vi "BrushedData (RT).vi"() -> ()   [LabVIEW 2013]
uses:
  <vilib>/FPGAPlugInAG/sbRIO-9626/niLvFpga_Open_sbRIO-9626.vi
  <vilib>/rvi/interface/common/dynamic/niFpgaDynamicAddResources.vi
  <vilib>/FPGAPlugInAG/Dynamic/niLvFpga_Reset_Dynamic.vi
  <vilib>/FPGAPlugInAG/Dynamic/niLvFpga_Run_Dynamic.vi
  <vilib>/rvi/interface/common/niFpgaWaitOnOcc.vi
  <vilib>/Utility/error.llb/Error Cluster From Error Code.vi
  <vilib>/rvi/errors/niLvFpgaAdjustHostInterfaceError.vi
  <vilib>/rvi/interface/nirviOpenFPGA/nirviOpenFPGA.xnode
  FPGA/bitfiles/TI sbRIO PWM (FPGA) v1.0.lvbitx
  <vilib>/rvi/interface/nirviMethod/nirviMethod.xnode
  <vilib>/rvi/interface/nirviReadWriteControl/nirviReadWriteControl.xnode
  <vilib>/FPGAPlugInAG/Dynamic/niLvFpga_ReadFifo_Dynamic.vi
  <vilib>/rvi/errors/niLvFpgaMergeErrorWithErrorCode.vi
  NiFpgaLv.dll
  <vilib>/rvi/interface/Simulation/niFpgaSimulationCallBeginRW.vi
panel:
  out "RPM2":dbl
  out "RPM1":dbl
  in  "hysteresis":fxp<+,25,6>=1.0
  in  "Stream":bool
  out "Pos2Currents":dbl[][](graph)
  out "Frequency":dbl[][](graph)
  out "Pos1Currents":dbl[][](graph)
  in  "StdFreqUpdt":bool
  in  "ReadData":bool
  in  "stop":bool
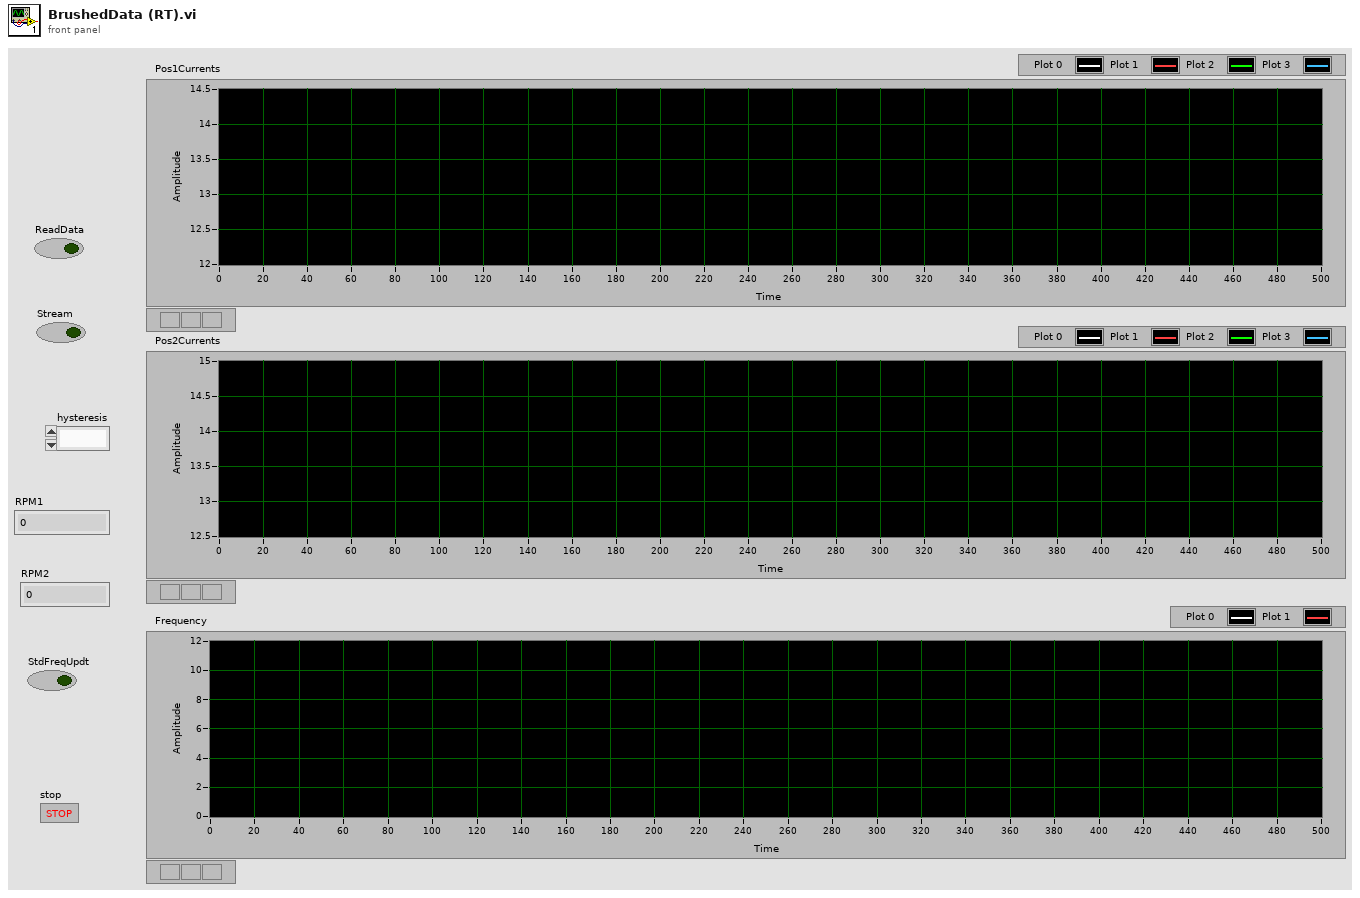
[diagram p1: front panel]
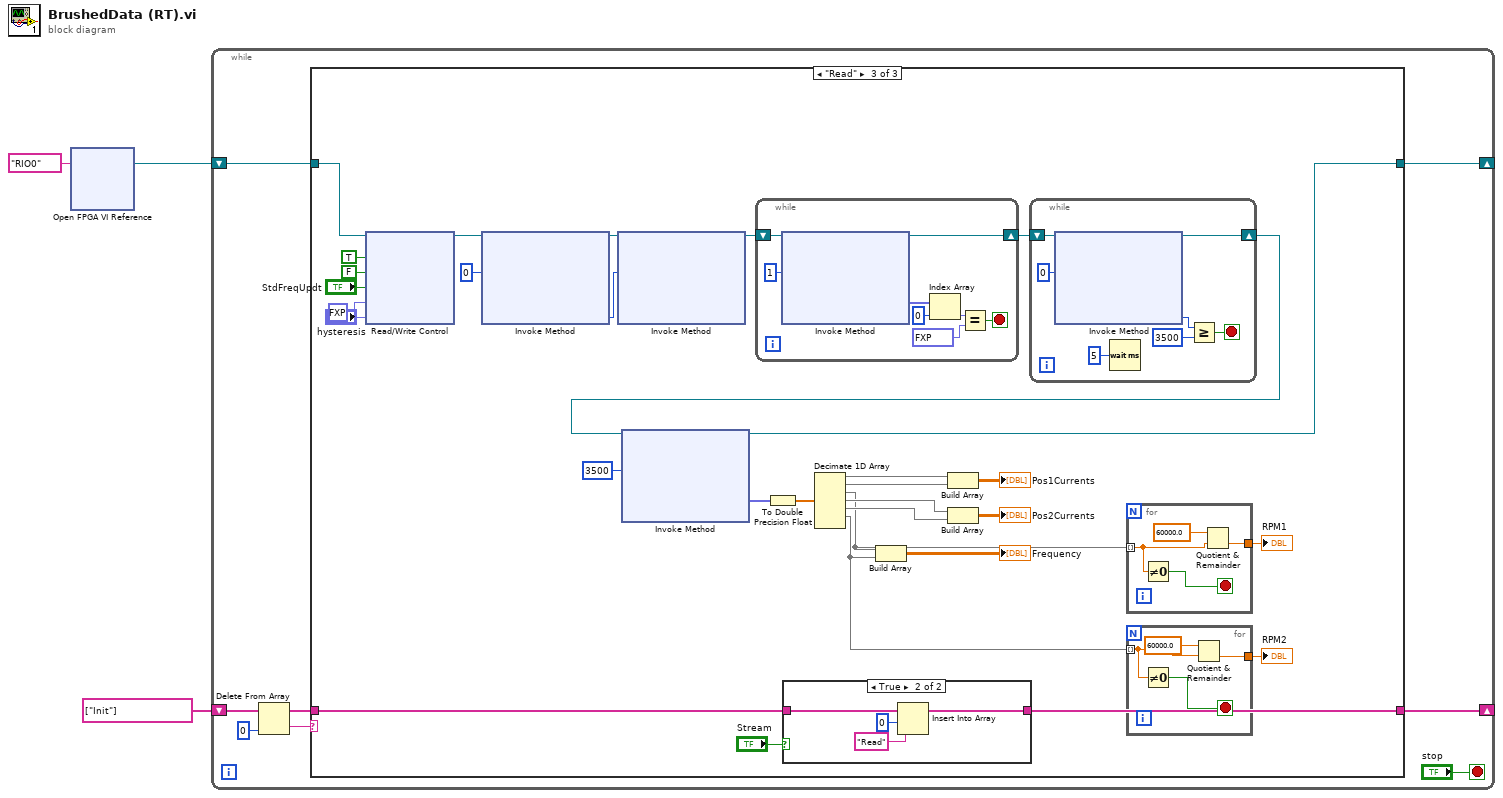
[diagram p0: block diagram]
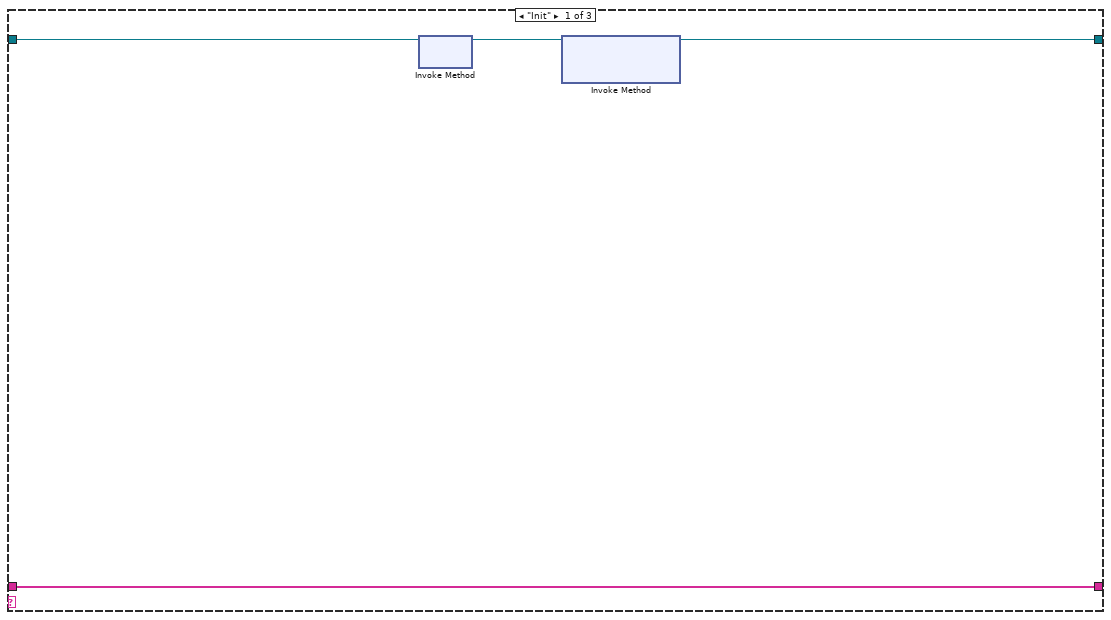
[diagram p2: hidden frame]
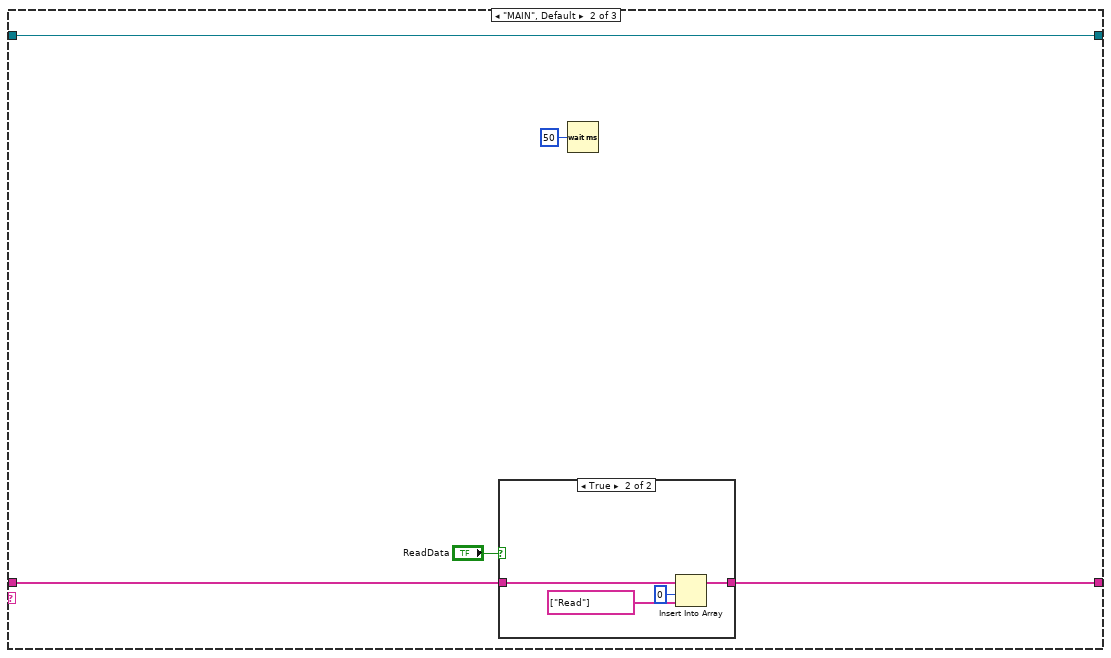
[diagram p3: hidden frame]
diagram:
  n1 = xnode "Open FPGA VI Reference"("resource name"=tag "RIO0") -> ("FPGA VI Reference Out"=w2:refnum<k20>)  [unwired: 1 in, 1 out]
  n2 = while {
    shift-right: [w6] -> _
    shift-left: string[] ["Init"] -> [w10]
    shift-right: [w5] -> _
    shift-left: w2 -> [w4]
    stop <- "stop" stop-if-true
    n3 = Delete From Array(array=w10, index=0) -> (deleted portion=w8:string, array with subset deleted=w7:string[])  [unwired: 1 in]
    n4 = case shown="\"Read\"" w8 {
      tunnel: w7 -> [w12 w17 w33]
      tunnel: [w12 w16 w32] -> w6
      tunnel: w4 -> [w15 w20 w56]
      tunnel: [w13 w20 w42] -> w5
      frame "Init" {
        n5 = xnode "Invoke Method"("FPGA VI Reference In"=w15) -> ("FPGA VI Reference Out"=w14:refnum<k20>)  [unwired: 1 in, 1 out]
        n6 = xnode "Invoke Method"("FPGA VI Reference In"=w14) -> ("FPGA VI Reference Out"=w13:refnum<k20>)  [unwired: 2 in, 1 out]
      }
      frame "MAIN", Default {
        n7 = case shown="True" "ReadData" {
          tunnel: w17 -> [w21 w25]
          tunnel: [w21 w24] -> w16
          frame False {
          }
          frame True {
            n8 = Insert Into Array(array=w25, index=0, new element=string[] ["Read"]) -> (w24:string[])
          }
        }
        n9 = Wait (ms)(milliseconds to wait=u32 50) -> ()  [unwired: 1 out]
      }
      frame "Read" {
        n10 = xnode "Read/Write Control"("FPGA VI Reference In"=w56, "DIO63"=TRUE, "Brushless"=FALSE, "StdFreqUpdt"="StdFreqUpdt", "CommFactor"=fxp<+,32,16> 5.0, "hysteresis"="hysteresis") -> ("FPGA VI Reference Out"=w48:refnum<k20>)  [unwired: 1 in, 1 out]
        n11 = xnode "Invoke Method"("FPGA VI Reference In"=w48, "Number of Elements"=u32 0) -> ("FPGA VI Reference Out"=w47:refnum<k20>, "Elements Remaining"=w44:u32)  [unwired: 2 in, 2 out]
        n12 = xnode "Invoke Method"("FPGA VI Reference In"=w47, "Number of Elements"=w44) -> ("FPGA VI Reference Out"=w46:refnum<k20>)  [unwired: 2 in, 3 out]
        n13 = while {
          shift-right: [w81] -> w55
          shift-left: w46 -> [w82]
          stop <- w83 stop-if-true
          n14 = xnode "Invoke Method"("FPGA VI Reference In"=w82, "Number of Elements"=u32 1) -> ("FPGA VI Reference Out"=w81:refnum<k20>, "Data"=w79:fxp<+/-,32,16>[])  [unwired: 2 in, 2 out]
          n15 = Index Array(array=w79, index=0) -> (element=w77:fxp<+/-,32,16>)
          n16 = Equal?(x=w77, y=fxp<+/-,32,16> -32768.0) -> (x = y?=w83:bool)
        }
        n17 = case shown="True" "Stream" {
          tunnel: w33 -> [w65 w69]
          tunnel: [w65 w68] -> w32
          frame False {
          }
          frame True {
            n18 = Insert Into Array(array=w69, index=0, new element="Read" ("new element/subarray")) -> (w68:string[])
          }
        }
        n19 = while {
          shift-right: [w73] -> w43
          shift-left: w55 -> [w74]
          stop <- w75 stop-if-true
          n20 = xnode "Invoke Method"("FPGA VI Reference In"=w74, "Number of Elements"=u32 0) -> ("FPGA VI Reference Out"=w73:refnum<k20>, "Elements Remaining"=w71:u32)  [unwired: 2 in, 2 out]
          n21 = Wait (ms)(milliseconds to wait=u32 5) -> ()  [unwired: 1 out]
          n22 = Greater Or Equal?(x=w71, y=u32 3500) -> (x >= y?=w75:bool)
        }
        n23 = xnode "Invoke Method"("FPGA VI Reference In"=w43, "Number of Elements"=u32 3500) -> ("FPGA VI Reference Out"=w42:refnum<k20>, "Data"=w40:fxp<+/-,32,16>[])  [unwired: 2 in, 2 out]
        n24 = To Double Precision Float(number=w40) -> (double precision float=w54:dbl[])
        n25 = Decimate 1D Array(w54) -> (w53:dbl[], w36:dbl[], w29:dbl[], w35:dbl[], w34:dbl[], w28:dbl[])  [unwired: 1 out]
        n26 = Build Array(w29, w28) -> (→"Frequency":dbl[][])
        n27 = Build Array(w53, w36) -> (→"Pos1Currents":dbl[][])
        n28 = Build Array(w35, w34) -> (→"Pos2Currents":dbl[][])
        n29 = for {
          tunnel: w29 -> [w62] mode=indexing
          tunnel: [w61] -> w27
          stop <- w64 stop-if-true
          n30 = Not Equal To 0?(x=w62) -> (x != 0?=w64:bool)
          n31 = Quotient & Remainder(x=60000.0, y=w62) -> (floor(x/y)=w61:dbl)  [unwired: 1 out]
        }
        "RPM1" <- w27
        n32 = for {
          tunnel: w28 -> [w59] mode=indexing
          tunnel: [w57] -> w26
          stop <- w60 stop-if-true
          n33 = Not Equal To 0?(x=w59) -> (x != 0?=w60:bool)
          n34 = Quotient & Remainder(x=60000.0, y=w59) -> (floor(x/y)=w57:dbl)  [unwired: 1 out]
        }
        "RPM2" <- w26
      }
    }
  }
